vi "get_header.vi"(11 "all rows":string[][](array[string])) -> (3 "header":T1)   [LabVIEW 2019]
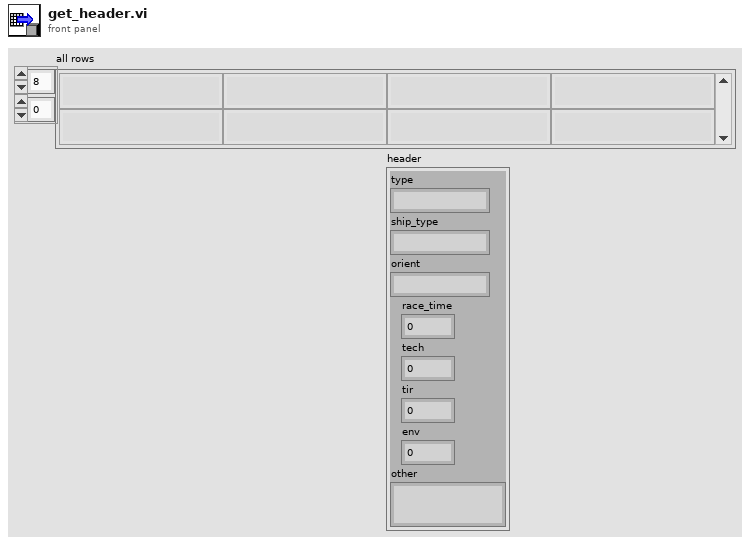
[diagram p1: front panel]
types:
  T1 = cluster{"type":string, "ship_type":string, "orient":string, "race_time":dbl, "tech":dbl, "tir":dbl, "env":dbl, "other":string}
  T2 = cluster{"type":string, "ship_type":string, "orient":string, "race_time":dbl, "tech":i32, "tir":i32, "env":i32, "other":string}
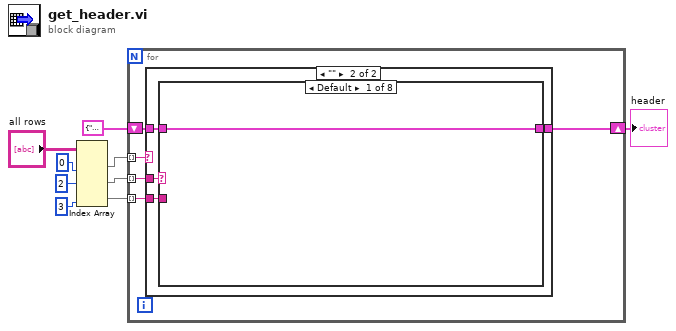
[diagram p0: block diagram]
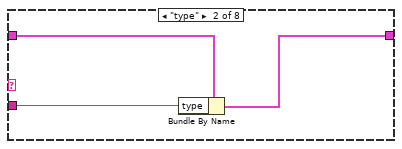
[diagram p3: hidden frame]
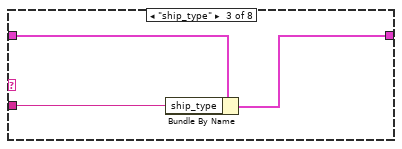
[diagram p4: hidden frame]
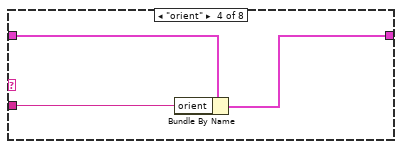
[diagram p5: hidden frame]
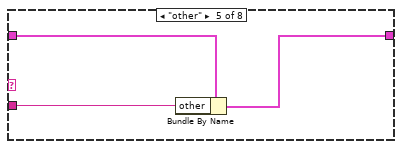
[diagram p6: hidden frame]
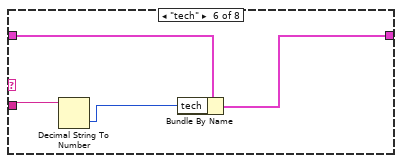
[diagram p7: hidden frame]
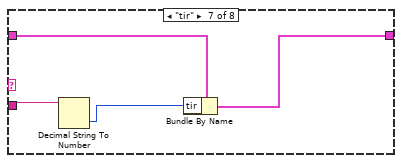
[diagram p8: hidden frame]
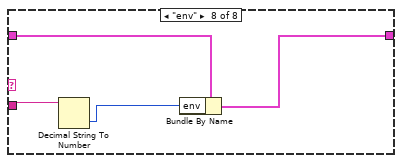
[diagram p9: hidden frame]
diagram:
  n1 = Index Array(array="all rows", index (col) #1=0 ("disabled index (col)"), index (col) #2=2 ("disabled index (row)"), index (col) #3=3 ("disabled index (row)")) -> (element #1=w8:string[], element #2=w7:string[], element #3=w6:string[])  [unwired: 3 in]
  n2 = for {
    tunnel: w8 -> [w14] mode=indexing
    tunnel: w7 -> [w13] mode=indexing
    tunnel: w6 -> [w12] mode=indexing
    shift-right: [w11] -> w4
    shift-left: T2 {"type"="", "ship_type"="", "orient"="", "race_time"=0.0, "tech"=0, "tir"=0, "env"=0, "other"=""} -> [w10]
    n3 = case shown="\"\"" w14 {
      tunnel: w13 -> [_ w19]
      tunnel: w12 -> [_ w18]
      tunnel: [w15 w17] -> w11
      tunnel: w10 -> [w15 w16]
      frame Default {
      }
      frame "" {
        n4 = case shown="Default" w19 {
          tunnel: w18 -> [_ w23 w26 w29 w32 w34 w38 w42]
          tunnel: [w20 w22 w25 w28 w31 w36 w40 w44] -> w17
          tunnel: w16 -> [w20 w21 w24 w27 w30 w35 w39 w43]
          frame Default {
          }
          frame "type" {
            n5 = Bundle By Name(cluster=w21, "type"=w23) -> (w22:T2)
          }
          frame "ship_type" {
            n6 = Bundle By Name(cluster=w24, "ship_type"=w26) -> (w25:T2)
          }
          frame "orient" {
            n7 = Bundle By Name(cluster=w27, "orient"=w29) -> (w28:T2)
          }
          frame "other" {
            n8 = Bundle By Name(cluster=w30, "other"=w32) -> (w31:T2)
          }
          frame "tech" {
            n9 = Decimal String To Number(string=w34) -> (number=w33:i32)  [unwired: 2 in, 1 out]
            n10 = Bundle By Name(cluster=w35, "tech"=w33) -> (w36:T2)
          }
          frame "tir" {
            n11 = Decimal String To Number(string=w38) -> (number=w37:i32)  [unwired: 2 in, 1 out]
            n12 = Bundle By Name(cluster=w39, "tir"=w37) -> (w40:T2)
          }
          frame "env" {
            n13 = Decimal String To Number(string=w42) -> (number=w41:i32)  [unwired: 2 in, 1 out]
            n14 = Bundle By Name(cluster=w43, "env"=w41) -> (w44:T2)
          }
        }
      }
    }
  }
  "header" <- w4
